vi "AngularChange.vi"(1 "Degrees":dbl[](array[numeric]) format="%7.2f", 2 "Time":i32) -> (0 "Angular Change":dbl)   [LabVIEW 2009]
doc: "Uses unitialized shift registers to maintain a brief history of the joint angles and the times at which they occured. Uses this to determine a single indicator of joint change overall in the hand."
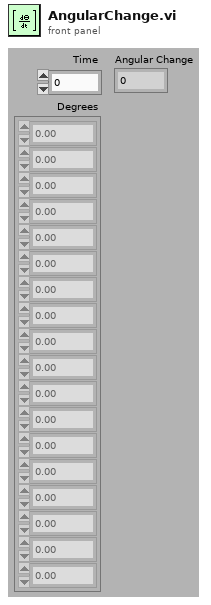
[diagram p1: front panel]
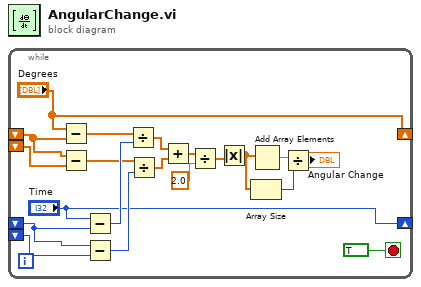
[diagram p0: block diagram]
diagram:
  n1 = while {
    shift-right: ["Time"] -> _
    shift-left: _ -> [w9]
    shift-right: ["Degrees"] -> _
    shift-left: _ -> [w6]
    shift-left: _ -> [w5]
    shift-left: _ -> [w8]
    stop <- TRUE stop-if-true
    n2 = Subtract(x="Degrees", y=w6) -> (x-y=w4:dbl[])
    n3 = Subtract(x=w6, y=w5) -> (x-y=w3:dbl[])
    n4 = Subtract(x="Time", y=w9) -> (x-y=w15:i32)
    n5 = Subtract(x=w9, y=w8) -> (x-y=w14:i32)
    n6 = Divide(x=w4, y=w15) -> (x/y=w13:dbl[])
    n7 = Divide(x=w3, y=w14) -> (x/y=w12:dbl[])
    n8 = Add(x=w13, y=w12) -> (x+y=w19:dbl[])
    n9 = Divide(x=w19, y=2.0 ("Degrees")) -> (x/y=w2:dbl[])
    n10 = Absolute Value(x=w2) -> (abs(x)=w1:dbl[])
    n11 = Array Size(array=w1) -> (size(s)=w16:i32)
    n12 = Add Array Elements(numeric array=w1) -> (sum=w17:dbl)
    n13 = Divide(x=w17, y=w16) -> (x/y=→"Angular Change":dbl)
  }
